vi "analyze pyro readout.vi"(9 "low cutoff freq: fl":dbl=0.12500000000000006 format="%#_13g", 10 "readout":dbl[](array[numeric]), 11 "background":dbl[](array[numeric])) -> (2 "max value":dbl, 4 "filtered signal":dbl[](array[numeric]), 5 "signal integral":dbl)   [LabVIEW 2020, in "TCPClient.lvclass"]
uses:
  TCPClient.lvclass
  <vilib>/Analysis/2dsp.llb/Integral Method.ctl
  <vilib>/Analysis/3filter.llb/Filter Passband Type.ctl
  <vilib>/Analysis/baseanly.llb/Mean (DBL).vi
  <vilib>/Analysis/8numeric.llb/1D Numeric Integration.vi
  <vilib>/Analysis/3filter.llb/Butterworth Filter (DBL).vi
  <vilib>/Analysis/NI_AALBase.lvlib
  <vilib>/Analysis/NI_AALPro.lvlib
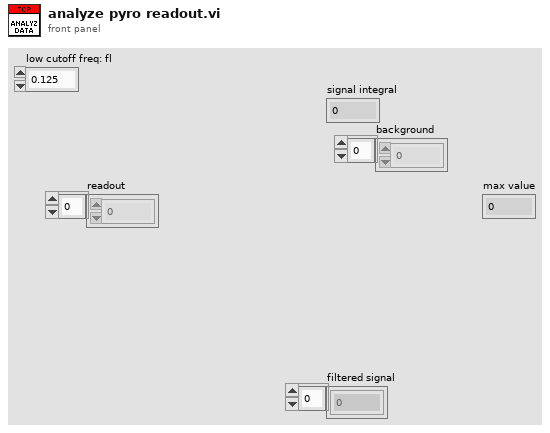
[diagram p1: front panel]
types:
  T1 = typedef "NI_AALBase.lvlib/Filter Passband Type.ctl" = enum32{"Lowpass", "Highpass", "Bandpass", "Bandstop"}
  T2 = typedef "NI_AALPro.lvlib/Integral Method.ctl" = i32
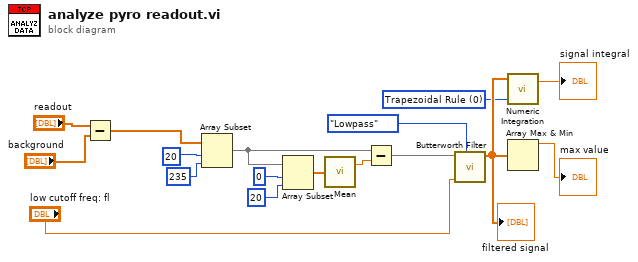
[diagram p0: block diagram]
diagram:
  w11 = T2 0 items=["Trapezoidal Rule", "Simpson's Rule", "Simpson's 3/8 Rule", "Bode Rule"] ("integration method")
  n1 = Subtract(x="readout", y="background") -> (x-y=w1:dbl[])
  n2 = Array Subset(array=w1, index=20, length=235) -> (w9:dbl[])
  n3 = Array Subset(array=w9, index=0, length=20) -> (w8:dbl[])
  n4 = call-poly <vilib>:"Mean.vi"("X"=w8) -> ("mean"=w10:dbl)  [unwired: 1 out]
  n5 = Subtract(x=w9, y=w10) -> (x-y=w14:dbl[])
  n6 = call-poly <vilib>:"Butterworth Filter.vi"("filter type"=Filter_Passband_Type."Lowpass", "low cutoff freq: fl"="low cutoff freq: fl", "X"=w14) -> ("Filtered X"=w17:dbl[])  [unwired: 5 in, 1 out]
  "filtered signal" <- w17
  n7 = call-poly <vilib>:"Numeric Integration.vi"("integration method"=w11, "Input Array"=w17) -> ("result"=→"signal integral":dbl)  [unwired: 1 in, 1 out]
  n8 = Array Max & Min(array=w17) -> (max value=→"max value":dbl)  [unwired: 3 out]
